vi "Build Module Map.vi"(8 "error in (no error)":errorcluster, 11 "DAQmxDI in":refnum<class "DAQmxDI.lvclass">) -> (0 "error out":errorcluster, 2 "Channels":string[](array[string]), 3 "DAQmxDI out":refnum<class "DAQmxDI.lvclass">)   [LabVIEW 2020, in "VolatusDAQ.lvlib" / "DAQmxDI.lvclass"]
uses:
  DAQmxDI.lvclass
  C:/dev/lv20CE/relink/lv-volatus/Volatus/Module/Module.lvclass
  Volatus/Event Level.ctl
  DAQmxDI.lvclass/DAQmxDI.ctl
  Volatus/Module/Module.lvclass/Module.ctl
  VolatusConfig/VolatusConfigElement/VolatusConfigElement.lvclass/VolatusConfigElement.ctl
  <vilib>/Utility/miscctls.llb/LVMapReplaceAction.ctl
  Volatus/Module/Config.vi
  VolatusConfig/VolatusConfigElement/Lookup Child by Name.vi
  VolatusConfig/VolatusConfigElement/Element.vi
  VolatusConfig/Channel/Channel Config.lvclass
  C:/dev/lv20CE/relink/lv-volatus/VolatusConfig/VolatusConfigElement/VolatusConfigElement.lvclass
  lv-cdm/CDM-Config/Config Element/Lookup Child by Name.vi
  lv-cdm/CDM-Config/Config Element/Value (String).vi
  VolatusConfig/Task/Task Config.lvclass
  Volatus/Module/Module.lvclass
  Volatus/Volatus.lvlib
  VolatusConfig/Group/Group Config.lvclass
  VolatusConfig/VolatusConfigElement/VolatusConfigElement.lvclass
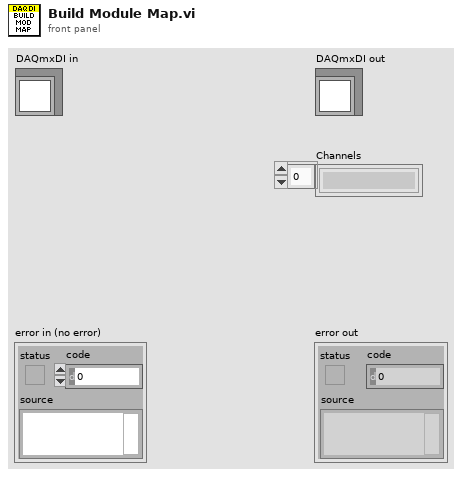
[diagram p1: front panel]
types:
  T1 = typedef "Volatus.lvlib/Event Level.ctl" = enum16{"Debug", "Info", "Warning", "Error"}
  T2 = typedef "VolatusDAQ.lvlib/DAQmxDI.lvclass/Port Info.ctl" = cluster{"Module Alias":string, "Number":i32, "# Lines":i32, "Lines":map{i32, string}, "Channel Indices":i32[]}
  T3 = typedef "VolatusDAQ.lvlib/DAQmxDI.lvclass/Digital Line.ctl" = cluster{"Module Alias":string, "Port":i32, "Line":i32}
  T4 = typedef "LVMapReplaceAction.ctl" = enum32{"Modify Entry only if found", "Add or Modify Entry", "Delete Entry"}
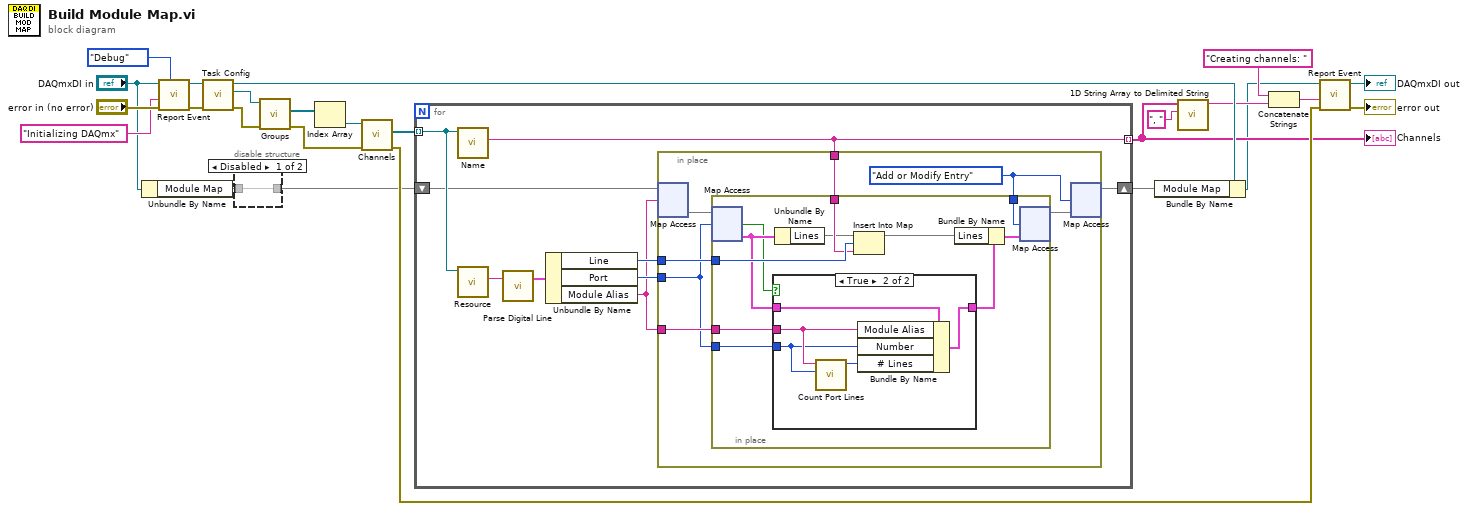
[diagram p0: block diagram]
diagram:
  n1 = Unbundle By Name("DAQmxDI in") -> ("Module Map"=w4:map{string, map{i32, T2}})
  n2 = call "Report Event.vi"("Level (Info)"=Event_Level."Debug", "error in (no error)"="error in (no error)", "Message"="Initializing DAQmx", "Module in"="DAQmxDI in") -> ("error out"=w18:errorcluster, "Module out"=w17:refnum<class "DAQmxDI.lvclass">)  [unwired: 6 in]
  n3 = call "Task Config.vi"("error in (no error)"=w18, "Module in"=w17) -> ("error out"=w23:errorcluster, "Task Config"=w22:refnum<class "Task Config.lvclass">, "Module out"=w20:refnum<class "DAQmxDI.lvclass">)  [unwired: 7 in]
  n4 = disable-structure shown="Disabled" {
    disable-tunnel: [w26 _] -> w5
    disable-tunnel: w4 -> [w26 _]
    frame Disabled {
    }
    frame Enabled {
    }
  }
  n5 = call "Groups.vi"("error in (no error)"=w23, "Task in"=w22) -> ("error out"=w3:errorcluster, "Groups"=w21:refnum<class "Group Config.lvclass">[])  [unwired: 7 in, 1 out]
  n6 = Index Array(array=w21) -> (element=w19:refnum<class "Group Config.lvclass">)  [unwired: 1 in]
  n7 = call "Channels.vi"("error in (no error)"=w3, "Group in"=w19) -> ("error out"=w25:errorcluster, "Channels"=w10:refnum<class "Channel Config.lvclass">[])  [unwired: 7 in, 1 out]
  n8 = for {
    tunnel: w10 -> [w35] mode=indexing
    tunnel: [w29] -> w9 mode=indexing
    shift-right: [w28] -> w1
    shift-left: w5 -> [w32]
    n9 = call "Name.vi"("VolatusConfigElement in"=w35) -> ("Name"=w29:string)  [unwired: 8 in, 2 out]
    n10 = call "Resource.vi"("Channel in"=w35) -> ("Resource"=w34:string)  [unwired: 8 in, 2 out]
    n11 = call "Parse Digital Line.vi"("Resource String"=w34) -> ("Digital Channel"=w33:T3)  [unwired: 6 in]
    n12 = Unbundle By Name(w33) -> ("Line"=w30:i32, "Port"=w31:i32, "Module Alias"=w27:string)
    n13 = in-place {
      in-place-border: w31 -> [w37]
      in-place-border: w30 -> [w40]
      in-place-border: w29 -> [w39]
      in-place-border: w27 -> [w38]
      w36 = LVMapReplaceAction."Add or Modify Entry" ("action")
      n14 = in-place-map #1(w32, w27) -> (w42:map{i32, T2})  [unwired: 1 in, 1 out]
      n15 = in-place {
        in-place-border: w40 -> [w53]
        in-place-border: w39 -> [w52]
        in-place-border: w38 -> [w48]
        in-place-border: w37 -> [w47]
        in-place-border: w36 -> [w43]
        n16 = in-place-map #2(w42, w37) -> (w50:T2, w49:bool)  [unwired: 1 in]
        n17 = case shown="True" w49 {
          tunnel: w50 -> [w54 w59]
          tunnel: w48 -> [_ w56]
          tunnel: w47 -> [_ w55]
          tunnel: [w54 w58] -> w46
          frame False {
          }
          frame True {
            n18 = call "Count Port Lines.vi"("Port"=w55, "ActiveDev"=w56) -> ("# Lines"=w57:i32)  [unwired: 9 in]
            n19 = Bundle By Name(cluster=w59, "Module Alias"=w56, "Number"=w55, "# Lines"=w57) -> (w58:T2)
          }
        }
        n20 = Unbundle By Name(w50) -> ("Lines"=w51:map{i32, string})
        n21 = Insert Into Map(map in=w51, key=w53, value=w52) -> (map out=w45:map{i32, string})  [unwired: 2 out]
        n22 = Bundle By Name(cluster=w46, "Lines"=w45) -> (w44:T2)
        n23 = in-place-map #2(w44, w43) -> (w41:map{i32, T2})  [unwired: 2 out]
      }
      n24 = in-place-map #1(w41, w36) -> (w28:map{string, map{i32, T2}})  [unwired: 2 out]
    }
  }
  "Channels" <- w9
  n25 = Bundle By Name(cluster=w20, "Module Map"=w1) -> (w2:refnum<class "DAQmxDI.lvclass">)
  n26 = call <vilib>:"1D String Array to Delimited String.vi"("delimiter"=", ", "string array"=w9) -> ("delimited string"=w12:string)  [unwired: 9 in]
  n27 = Concatenate Strings("Creating channels: " ("Message"), w12) -> (w11:string)
  n28 = call "Report Event.vi"("error in (no error)"=w25, "Message"=w11, "Module in"=w2) -> ("error out"=→"error out":errorcluster, "Module out"=→"DAQmxDI out":refnum<class "DAQmxDI.lvclass">)  [unwired: 7 in]
